vi "SMC.vi"() -> ()   [LabVIEW 2010]
doc: "This is the Superconducting Magnet Control module (SMC).\nIts job is to receive messages from the PDP, translate them into magnet commands, and send reply messages back to the PDP indicating magnet status."
uses:
  SMC Global.vi
panel:
  in  "Force Read":bool
  in  "Need to Beep":bool
  in  "Beep at Setpoint":bool=TRUE
  out "SMC Message Type":T1(ring)=enum."Ping="
  out "Magnet Entered this state at:":string
  out "Last Change":dbl format="%.2f"
  out "Update Often":bool
  out "Magnet Status":T2={"Sweep Status"=enum."To Zero", "Leads Current (A)"=0.0, "Leads Voltage (V)"=0.0, "Leads Field (T)"=0.0, "Switch Heater"=FALSE, "Setpoint (A)"=0.0, "Sweep Rate (A/min)"=0.0, "System Status"=enum."Warming Up", "Limit Status"=enum."Positive Current Limit", "Persistent Current (A)"=0.0, "Control Status"=FALSE, "Persistent Field (T)"=0.0} {"Leads Field (T)" format="%.2f"; "Persistent Field (T)" format="%.3f"; "Persistent Current (A)" format="%.3f"; "Setpoint (A)" format="%.3f"; "Leads Voltage (V)" format="%.2f"; "Sweep Rate (A/min)" format="%.2f"; "Leads Current (A)" format="%.3f"}
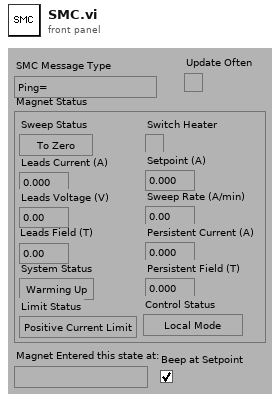
[diagram p1: front panel]
types:
  T1 = enum16{"Bad Message", "DoNothing", "Read=", "GenEvent=", "MagStatus=", "Control", "Setpoint=", "Setrate=", "Heater=", "Ping=", "Stop", "Beep"}
  T2 = cluster{"Sweep Status":enum16{"Hold", "To Setpoint", "To Zero", "Clamped"}, "Leads Current (A)":dbl, "Leads Voltage (V)":dbl, "Leads Field (T)":dbl, "Switch Heater":bool, "Setpoint (A)":dbl, "Sweep Rate (A/min)":dbl, "System Status":enum16{"Normal", "Quenched", "Over Heated", "Warming Up"}, "Limit Status":enum16{"Normal", "Positive Voltage Limit", "Negative Voltage Limit", "Negative Current Limit", "Positive Current Limit"}, "Persistent Current (A)":dbl, "Control Status":bool, "Persistent Field (T)":dbl}
  T3 = enum16{"Hold", "To Setpoint", "To Zero", "Clamped"}
  T4 = enum16{"Normal", "Quenched", "Over Heated", "Warming Up"}
  T5 = enum16{"Normal", "Positive Voltage Limit", "Negative Voltage Limit", "Negative Current Limit", "Positive Current Limit"}
  T6 = cluster{"Sweep Status":enum16{"Hold", "To Setpoint", "To Zero", "Clamped"}, "Leads Current (A)":dbl, "Leads Field (T)":dbl, "Switch Heater":bool, "Setpoint (A)":dbl, "Sweep Rate (A/min)":dbl, "System Status":enum16{"Normal", "Quenched", "Over Heated", "Warming Up"}, "Limit Status":enum16{"Normal", "Positive Voltage Limit", "Negative Voltage Limit", "Negative Current Limit", "Positive Current Limit"}, "Persistent Current (A)":dbl, "Control Status":bool, "Persistent Field (T)":dbl}
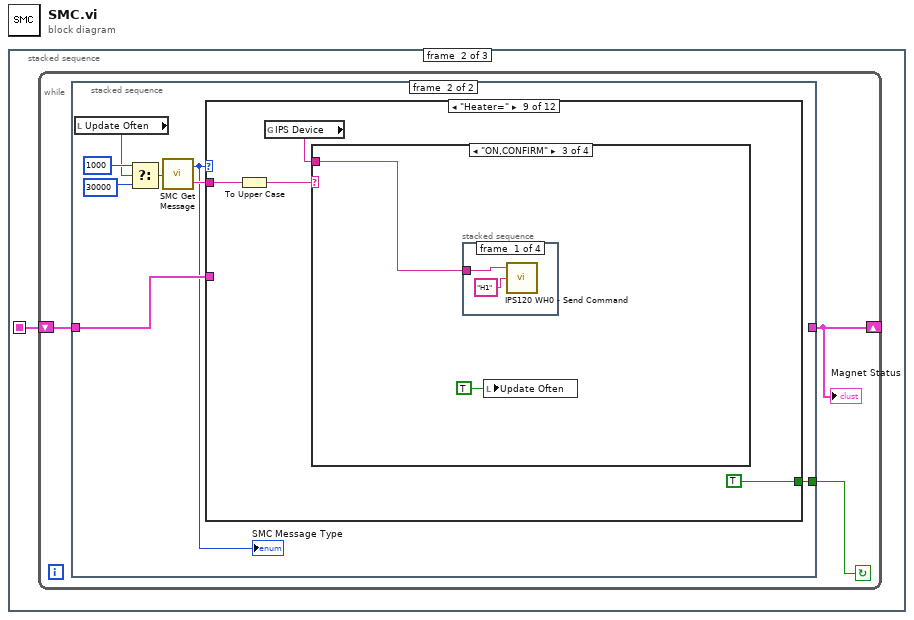
[diagram p0: block diagram]
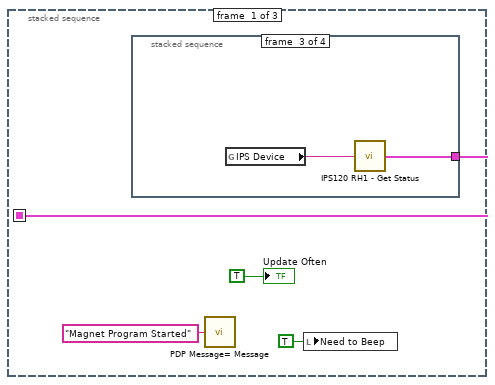
[diagram p2: hidden frame]
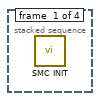
[diagram p3: hidden frame]
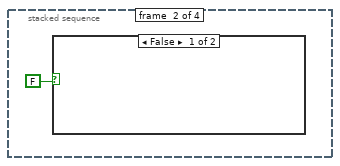
[diagram p4: hidden frame]
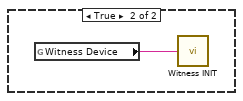
[diagram p5: hidden frame]
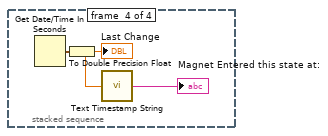
[diagram p6: hidden frame]
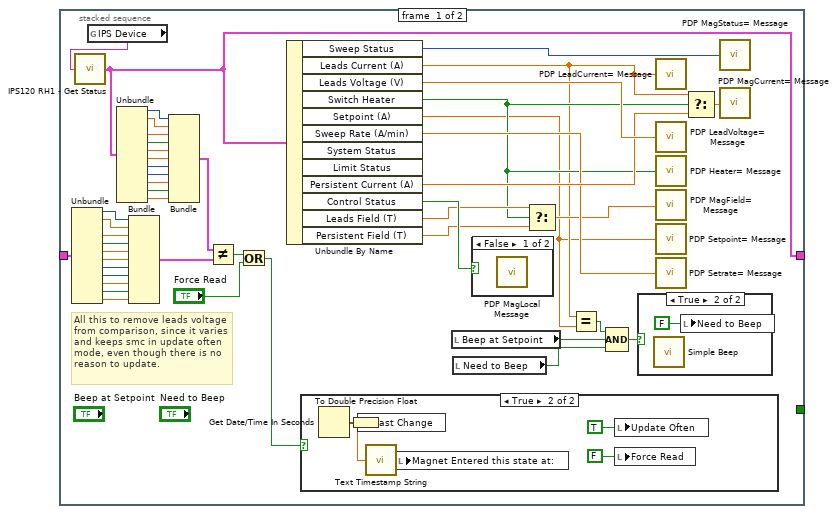
[diagram p7: hidden frame]
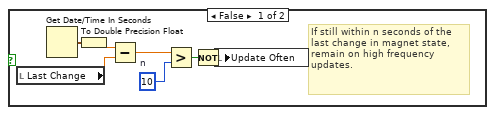
[diagram p8: hidden frame]
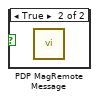
[diagram p10: hidden frame]
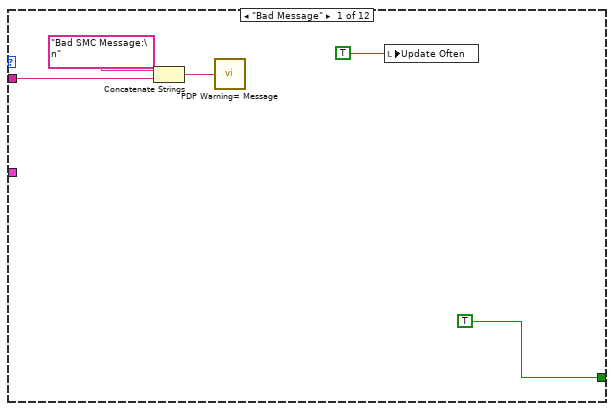
[diagram p11: hidden frame]
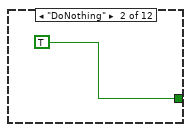
[diagram p12: hidden frame]
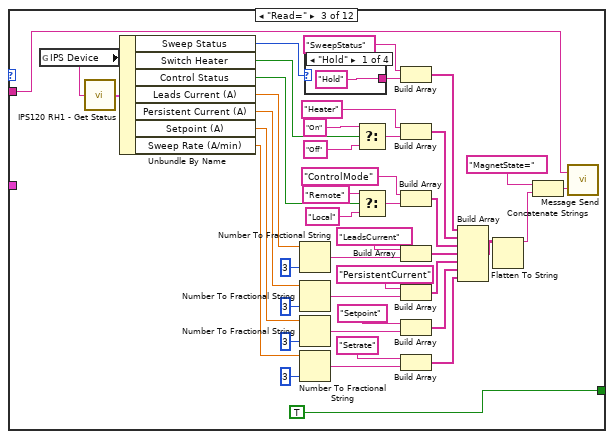
[diagram p13: hidden frame]
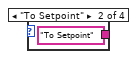
[diagram p14: hidden frame]
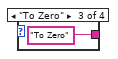
[diagram p15: hidden frame]
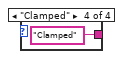
[diagram p16: hidden frame]
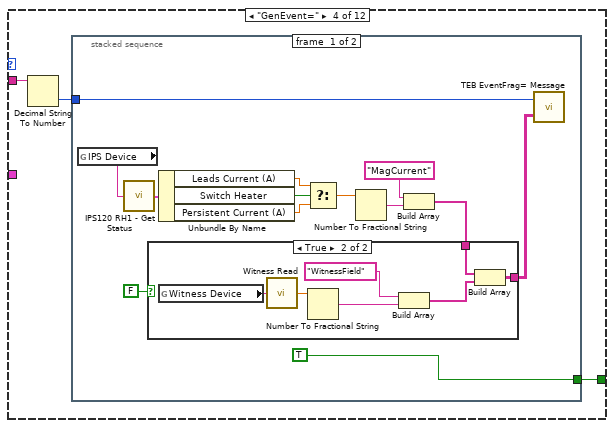
[diagram p17: hidden frame]
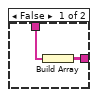
[diagram p18: hidden frame]
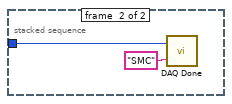
[diagram p19: hidden frame]
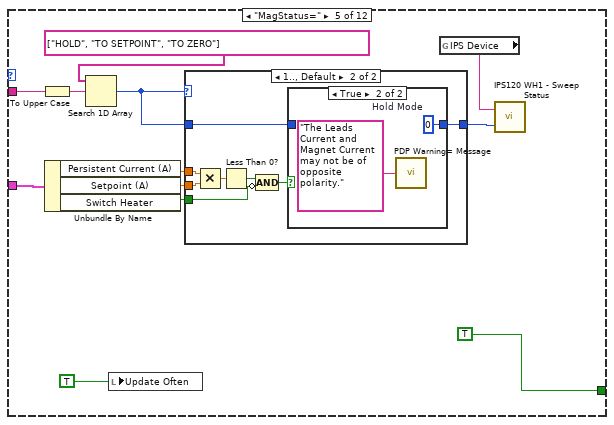
[diagram p20: hidden frame]
diagram:
  n1 = stacked-sequence {
    seq-local: [w4 _ _] -> [_ w12 _]
    frame #0 {
      n2 = stacked-sequence {
        tunnel: [_ _ w8 _] -> w4
        frame #0 {
          n3 = call "SMC INIT.vi"() -> ()  [unwired: 1 in]
        }
        frame #1 {
          n4 = case shown="False" FALSE {
            frame False {
            }
            frame True {
              n5 = global read "SMC Global.vi" "Witness Device"() -> (w6:string)
              n6 = call "Witness INIT.vi"("address string"=w6) -> ()
            }
          }
        }
        frame #2 {
          n7 = global read "SMC Global.vi" "IPS Device"() -> (w7:string)
          n8 = call "IPS120 RH1 - Get Status.vi"("GPIB Address"=w7) -> ("Magnet Status"=w8:T2)
        }
        frame #3 {
          n9 = Get Date/Time In Seconds() -> (seconds since 1Jan1904=w9:timestamp)
          n10 = To Double Precision Float(number=w9) -> (double precision float=w11:dbl)
          "Last Change" <- w11
          n11 = call "Text Timestamp String.vi"("Seconds"=w11) -> ("Timestamp String"=→"Magnet Entered this state at:":string)
        }
      }
      n12 = call "PDP Message= Message.vi"("Message"="Magnet Program Started") -> ()
      n13 = local write "Need to Beep"(TRUE ("Need to Beep")) -> ()
      "Update Often" <- TRUE ("Update Often")
    }
    frame #1 {
      n14 = while {
        shift-left: w12 -> [w14]
        shift-right: [w13] -> _
        stop <- w15 continue-if-true
        n15 = stacked-sequence {
          tunnel: [_ w81] -> w15
          tunnel: w14 -> [w60 w77]
          tunnel: [w46 _] -> w13
          frame #0 {
            # "All this to remove leads voltage from comparison, since it varies and keeps smc in update often mode, even though there is no \nreason to update."
            n16 = Unbundle(w60) -> ("Sweep Status"=w59:T3, "Leads Current (A)"=w58:dbl, "Leads Field (T)"=w57:dbl, "Switch Heater"=w56:bool, "Setpoint (A)"=w55:dbl, "Sweep Rate (A/min)"=w54:dbl, "System Status"=w53:T4, "Limit Status"=w52:T5, "Persistent Current (A)"=w43:dbl, "Control Status"=w42:bool, "Persistent Field (T)"=w41:dbl)  [unwired: 1 out]
            n17 = global read "SMC Global.vi" "IPS Device"() -> (w61:string)
            n18 = call "IPS120 RH1 - Get Status.vi"("GPIB Address"=w61) -> ("Magnet Status"=w46:T2)
            n19 = Unbundle(w46) -> ("Sweep Status"=w35:T3, "Leads Current (A)"=w36:dbl, "Leads Field (T)"=w37:dbl, "Switch Heater"=w38:bool, "Setpoint (A)"=w39:dbl, "Sweep Rate (A/min)"=w40:dbl, "System Status"=w51:T4, "Limit Status"=w50:T5, "Persistent Current (A)"=w49:dbl, "Control Status"=w48:bool, "Persistent Field (T)"=w47:dbl)  [unwired: 1 out]
            n20 = Bundle("Sweep Status"=w59, "Leads Current (A)"=w58, "Leads Field (T)"=w57, "Switch Heater"=w56, "Setpoint (A)"=w55, "Sweep Rate (A/min)"=w54, "System Status"=w53, "Limit Status"=w52, "Persistent Current (A)"=w43, "Control Status"=w42, "Persistent Field (T)"=w41) -> (w44:T6)  [unwired: 1 in]
            n21 = Bundle("Sweep Status"=w35, "Leads Current (A)"=w36, "Leads Field (T)"=w37, "Switch Heater"=w38, "Setpoint (A)"=w39, "Sweep Rate (A/min)"=w40, "System Status"=w51, "Limit Status"=w50, "Persistent Current (A)"=w49, "Control Status"=w48, "Persistent Field (T)"=w47) -> (w45:T6)  [unwired: 1 in]
            n22 = Not Equal?(x=w45, y=w44) -> (x != y?=w33:bool)
            n23 = Or(x=w33, y="Force Read") -> (x .or. y?=w16:bool)
            n24 = Unbundle By Name(w46) -> ("Sweep Status"=w32:T3, "Leads Current (A)"=w22:dbl, "Leads Voltage (V)"=w31:dbl, "Switch Heater"=w24:bool, "Setpoint (A)"=w21:dbl, "Sweep Rate (A/min)"=w28:dbl, "Persistent Current (A)"=w30:dbl, "Control Status"=w27:bool, "Leads Field (T)"=w26:dbl, "Persistent Field (T)"=w25:dbl)  [unwired: 2 out]
            n25 = case shown="True" w16 {
              frame False {
                w65 = 10  # n
                # "If still within n seconds of the last change in magnet state, remain on high frequency updates."
                n26 = local read "Last Change"() -> (w64:dbl)
                n27 = Get Date/Time In Seconds() -> (seconds since 1Jan1904=w62:timestamp)
                n28 = To Double Precision Float(number=w62) -> (double precision float=w63:dbl)
                n29 = Subtract(x=w63, y=w64) -> (x-y=w66:dbl)
                n30 = Greater?(x=w66, y=w65) -> (0:w67:bool)
                n31 = Not(x=w67) -> (.not. x?=w68:bool)
                n32 = local write "Update Often"(w68) -> ()
              }
              frame True {
                n33 = Get Date/Time In Seconds() -> (seconds since 1Jan1904=w69:timestamp)
                n34 = To Double Precision Float(number=w69) -> (double precision float=w72:dbl)
                n35 = local write "Last Change"(w72) -> ()
                n36 = call "Text Timestamp String.vi"("Seconds"=w72) -> ("Timestamp String"=w73:string)
                n37 = local write "Magnet Entered this state at:"(w73) -> ()
                n38 = local write "Update Often"(TRUE ("Update Often")) -> ()
                n39 = local write "Force Read"(FALSE ("Force Read")) -> ()
              }
            }
            n40 = local read "Beep at Setpoint"() -> (w19:bool)
            n41 = local read "Need to Beep"() -> (w18:bool)
            n42 = case shown="False" w27 {
              frame False {
                n43 = call "PDP MagLocal Message.vi"() -> ()  [unwired: 1 in]
              }
              frame True {
                n44 = call "PDP MagRemote Message.vi"() -> ()  [unwired: 1 in]
              }
            }
            n45 = Select(t=w26, s=w24, f=w25) -> (s? t:f=w23:dbl)
            n46 = Equal?(x=w22, y=w21) -> (x = y?=w20:bool)
            n47 = Compound Arithmetic op=AND(w20, w19, w18) -> (w17:bool)
            n48 = case shown="True" w17 {
              frame False {
              }
              frame True {
                n49 = call "Simple Beep.vi"() -> ()  [unwired: 1 in]
                n50 = local write "Need to Beep"(FALSE) -> ()
              }
            }
            n51 = call "PDP LeadCurrent= Message.vi"("Lead Current"=w22) -> ()
            n52 = call "PDP LeadVoltage= Message.vi"("Lead Voltage"=w31) -> ()
            n53 = call "PDP Heater= Message.vi"("Setrate"=w24) -> ()
            n54 = call "PDP MagField= Message.vi"("Mag Field"=w23) -> ()
            n55 = call "PDP Setpoint= Message.vi"("Setpoint"=w21) -> ()
            n56 = call "PDP Setrate= Message.vi"("Setrate"=w28) -> ()
            n57 = Select(t=w22, s=w24, f=w30) -> (s? t:f=w29:dbl)
            n58 = call "PDP MagStatus= Message.vi"("Mag Status"=w32) -> ()
            n59 = call "PDP MagCurrent= Message.vi"("Mag Current"=w29) -> ()
          }
          frame #1 {
            n60 = local read "Update Often"() -> (w75:bool)
            n61 = Select(t=1000, s=w75, f=30000) -> (s? t:f=w80:i32)
            n62 = call "SMC Get Message.vi"("Timeout (ms)"=w80) -> ("SMC Message Type"=w76:T1, "Text"=w82:string)
            "SMC Message Type" <- w76
            n63 = case shown="\"Heater=\"" w76 {
              tunnel: w82 -> [w87 _ w92 w138 w174 _ w196 w201 w205 w249 _ _]
              tunnel: [TRUE TRUE TRUE w139 TRUE TRUE TRUE TRUE TRUE TRUE FALSE TRUE] -> w81
              tunnel: w77 -> [_ _ _ _ w167 w191 _ _ _ _ _ _]
              frame "Bad Message" {
                n64 = Concatenate Strings("Bad SMC Message:\n", w87) -> (w85:string)
                n65 = call "PDP Warning= Message.vi"("Message"=w85) -> ()
                n66 = local write "Update Often"(TRUE) -> ()
              }
              frame "DoNothing" {
              }
              frame "Read=" {
                n67 = global read "SMC Global.vi" "IPS Device"() -> (w131:string)
                n68 = call "IPS120 RH1 - Get Status.vi"("GPIB Address"=w131) -> ("Magnet Status"=w130:T2)
                n69 = Unbundle By Name(w130) -> ("Sweep Status"=w110:T3, "Switch Heater"=w111:bool, "Control Status"=w107:bool, "Leads Current (A)"=w122:dbl, "Persistent Current (A)"=w123:dbl, "Setpoint (A)"=w124:dbl, "Sweep Rate (A/min)"=w125:dbl)
                n70 = Number To Fractional String(number=w122, precision (6)=i16 3) -> (F-format string=w121:string)  [unwired: 2 in]
                n71 = Number To Fractional String(number=w123, precision (6)=i16 3) -> (F-format string=w119:string)  [unwired: 2 in]
                n72 = Number To Fractional String(number=w124, precision (6)=i16 3) -> (F-format string=w118:string)  [unwired: 2 in]
                n73 = Number To Fractional String(number=w125, precision (6)=i16 3) -> (F-format string=w117:string)  [unwired: 2 in]
                n74 = case shown="\"Hold\"" w110 {
                  tunnel: ["Hold" "To Setpoint" "To Zero" "Clamped"] -> w102
                  frame "Hold" {
                  }
                  frame "To Setpoint" {
                  }
                  frame "To Zero" {
                  }
                  frame "Clamped" {
                  }
                }
                n75 = Select(t="On", s=w111, f="Off") -> (s? t:f=w105:string)
                n76 = Select(t="Remote", s=w107, f="Local") -> (s? t:f=w106:string)
                n77 = Build Array("SweepStatus", w102) -> (w96:string[])
                n78 = Build Array("Heater", w105) -> (w95:string[])
                n79 = Build Array("ControlMode", w106) -> (w94:string[])
                n80 = Build Array("LeadsCurrent", w121) -> (w97:string[])
                n81 = Build Array("PersistentCurrent", w119) -> (w98:string[])
                n82 = Build Array("Setpoint", w118) -> (w99:string[])
                n83 = Build Array("Setrate", w117) -> (w100:string[])
                n84 = Build Array(w96, w95, w94, w97, w98, w99, w100) -> (w93:string[][])
                n85 = Flatten To String(anything=w93) -> (data string=w90:string)  [unwired: 3 in, 2 out]
                n86 = Concatenate Strings("MagnetState=" ("Substring"), w90) -> (w91:string)
                n87 = call "Message Send.vi"("Message"=w91, "Destination"=w92) -> ()
              }
              frame "GenEvent=" {
                n88 = Decimal String To Number(string=w138) -> (number=w137:i32)  [unwired: 2 in, 1 out]
                n89 = stacked-sequence {
                  tunnel: [TRUE _] -> w139
                  tunnel: w137 -> [w151 w163]
                  frame #0 {
                    n90 = global read "SMC Global.vi" "IPS Device"() -> (w145:string)
                    n91 = call "IPS120 RH1 - Get Status.vi"("GPIB Address"=w145) -> ("Magnet Status"=w150:T2)
                    n92 = Unbundle By Name(w150) -> ("Leads Current (A)"=w143:dbl, "Switch Heater"=w144:bool, "Persistent Current (A)"=w142:dbl)
                    n93 = Select(t=w143, s=w144, f=w142) -> (s? t:f=w141:dbl)
                    n94 = Number To Fractional String(number=w141) -> (F-format string=w146:string)  [unwired: 3 in]
                    n95 = Build Array("MagCurrent", w146) -> (w148:string[])
                    n96 = case shown="True" FALSE {
                      tunnel: w148 -> [w154 w161]
                      tunnel: [w153 w160] -> w147
                      frame False {
                        n97 = Build Array(w154) -> (w153:string[][])
                      }
                      frame True {
                        n98 = global read "SMC Global.vi" "Witness Device"() -> (w155:string)
                        n99 = call "Witness Read.vi"("address string"=w155) -> ("Field"=w156:dbl)
                        n100 = Number To Fractional String(number=w156) -> (F-format string=w159:string)  [unwired: 3 in]
                        n101 = Build Array("WitnessField", w159) -> (w157:string[])
                        n102 = Build Array(w161, w157) -> (w160:string[][])
                      }
                    }
                    n103 = call "TEB EventFrag= Message.vi"("Event Fragment(s)"=w147, "Event Number"=w151) -> ()
                  }
                  frame #1 {
                    n104 = call "DAQ Done.vi"("Module Name"="SMC", "Event Number"=w163) -> ()
                  }
                }
              }
              frame "MagStatus=" {
                n105 = To Upper Case(1:w174) -> (0:w173:string)
                n106 = Unbundle By Name(w167) -> ("Persistent Current (A)"=w166:dbl, "Setpoint (A)"=w165:dbl, "Switch Heater"=w164:bool)
                n107 = Search 1D Array(1D array=string[] ["HOLD", "TO SETPOINT", "TO ZERO"], element=w173) -> (index of element=w169:i32)  [unwired: 1 in]
                n108 = local write "Update Often"(TRUE) -> ()
                n109 = case shown="1.., Default" w169 {
                  tunnel: w169 -> [w176 w181]
                  tunnel: w166 -> [_ w184]
                  tunnel: w165 -> [_ w183]
                  tunnel: [w176 w180] -> w168
                  tunnel: w164 -> [_ w178]
                  frame ..0 {
                  }
                  frame 1.., Default {
                    n110 = Multiply(x=w184, y=w183) -> (x*y=w182:dbl)
                    n111 = Less Than 0?(x=w182) -> (x < 0?=w179:bool)
                    n112 = Compound Arithmetic op=AND(w179, invert w178) -> (w177:bool)
                    n113 = case shown="True" w177 {
                      tunnel: w181 -> [w185 _]
                      tunnel: [w185 w187] -> w180
                      frame False {
                      }
                      frame True {
                        w187 = 0  # Hold Mode
                        n114 = call "PDP Warning= Message.vi"("Message"="The Leads Current and Magnet Current may not be of opposite polarity.") -> ()
                      }
                    }
                  }
                }
                n115 = global read "SMC Global.vi" "IPS Device"() -> (w172:string)
                n116 = call "IPS120 WH1 - Sweep Status.vi"("Sweep Status"=w168, "GPIB Address"=w172) -> ()
              }
              frame "Control" {
                n117 = global read "SMC Global.vi" "IPS Device"() -> (w188:string)
                n118 = Unbundle By Name(w191) -> ("Control Status"=w190:bool)
                n119 = Not(x=w190) -> (.not. x?=w189:bool)
                n120 = call "IPS120 WH4 - Remote Mode.vi"("Remote Mode"=w189, "GPIB Address"=w188) -> ()
              }
              frame "Setpoint=" {
                w193 = TRUE
                n121 = Fract/Exp String To Number(string=w196) -> (number=w195:dbl)  [unwired: 3 in, 1 out]
                n122 = global read "SMC Global.vi" "IPS Device"() -> (w194:string)
                n123 = call "IPS120 WH2 - Write Setpoint.vi"("Setpoint"=w195, "GPIB Address"=w194) -> ()
                n124 = local write "Update Often"(w193) -> ()
                n125 = local write "Need to Beep"(w193) -> ()
              }
              frame "Setrate=" {
                n126 = Fract/Exp String To Number(string=w201) -> (number=w200:dbl)  [unwired: 3 in, 1 out]
                n127 = global read "SMC Global.vi" "IPS Device"() -> (w199:string)
                n128 = call "IPS120 WH3 - Write Setrate.vi"("Setrate"=w200, "GPIB Address"=w199) -> ()
                n129 = local write "Update Often"(TRUE) -> ()
              }
              frame "Heater=" {
                n130 = To Upper Case(1:w205) -> (0:w203:string)
                n131 = global read "SMC Global.vi" "IPS Device"() -> (w204:string)
                n132 = case shown="\"ON,CONFIRM\"" w203 {
                  tunnel: w204 -> [w208 w218 w233 w240]
                  frame "OFF", Default {
                    n133 = call "IPS120 RH1 - Get Status.vi"("GPIB Address"=w208) -> ("Magnet Status"=w207:T2)
                    n134 = stacked-sequence {
                      tunnel: w208 -> [w211 _ _]
                      tunnel: w207 -> [_ w213 _]
                      frame #0 {
                        n135 = call "IPS120 WH0 - Send Command.vi"("Command String"="H0", "VISA Address"=w211) -> ()  [unwired: 1 in, 3 out]
                      }
                      frame #1 {
                        # "If heater was on, wait 30 sec for it to go off."
                        n136 = Unbundle By Name(w213) -> ("Switch Heater"=w212:bool)
                        n137 = case shown="True" w212 {
                          frame False {
                          }
                          frame True {
                            n138 = stacked-sequence {
                              frame #0 {
                                n139 = call "PDP HeaterDelay= Message.vi"("Setrate"=i8 30 ("Heater Delay (sec)")) -> ()
                              }
                              frame #1 {
                                n140 = Wait (ms)(milliseconds to wait=u32 30000) -> ()  [unwired: 1 out]
                              }
                            }
                          }
                        }
                      }
                      frame #2 {
                        n141 = call "PDP Heater= Message.vi"("Setrate"=FALSE ("Switch Heater")) -> ()
                      }
                    }
                    n142 = local write "Update Often"(TRUE) -> ()
                  }
                  frame "ON" {
                    n143 = call "IPS120 RH1 - Get Status.vi"("GPIB Address"=w218) -> ("Magnet Status"=w225:T2)
                    n144 = Unbundle By Name(w225) -> ("Sweep Status"=w223:T3, "Leads Current (A)"=w222:dbl, "Persistent Current (A)"=w221:dbl)
                    n145 = Equal?(x=T3."Hold" ("Sweep Status"), y=w223) -> (x = y?=w217:bool)
                    n146 = Equal?(x=w222, y=w221) -> (x = y?=w219:bool)
                    n147 = Compound Arithmetic op=AND(w217, w219) -> (w220:bool)
                    n148 = case shown="True" w220 {
                      tunnel: w219 -> [w229 _]
                      tunnel: w218 -> [_ _]
                      frame False {
                        n149 = Select(t="The Magnet Power Supply needs to be in Hold Mode.", s=w229, f="The Magnet Leads do not match the current in the magnet.") -> (s? t:f=w226:string)
                        n150 = call "PDP Warning= Message.vi"("Message"=w226) -> ()
                      }
                      frame True {
                        n151 = call "Message Send.vi"("Message"="HeaterDialog", "Destination"="PDP") -> ()
                      }
                    }
                  }
                  frame "ON,CONFIRM" {
                    n152 = stacked-sequence {
                      tunnel: w233 -> [w235 _ _ _]
                      frame #0 {
                        n153 = call "IPS120 WH0 - Send Command.vi"("Command String"="H1", "VISA Address"=w235) -> ()  [unwired: 1 in, 3 out]
                      }
                      frame #1 {
                        n154 = call "PDP HeaterDelay= Message.vi"("Setrate"=i8 30 ("Heater Delay (sec)")) -> ()
                      }
                      frame #2 {
                        n155 = Wait (ms)(milliseconds to wait=u32 30000) -> ()  [unwired: 1 out]
                      }
                      frame #3 {
                        n156 = call "PDP Heater= Message.vi"("Setrate"=TRUE ("Switch Heater")) -> ()
                      }
                    }
                    n157 = local write "Update Often"(TRUE) -> ()
                  }
                  frame "ON,FORCE" {
                    n158 = stacked-sequence {
                      tunnel: w240 -> [w242 _ _ _]
                      frame #0 {
                        n159 = call "IPS120 WH0 - Send Command.vi"("Command String"="H1", "VISA Address"=w242) -> ()  [unwired: 1 in, 3 out]
                      }
                      frame #1 {
                        n160 = call "PDP HeaterDelay= Message.vi"("Setrate"=i8 30 ("Heater Delay (sec)")) -> ()
                      }
                      frame #2 {
                        n161 = Wait (ms)(milliseconds to wait=u32 30000) -> ()  [unwired: 1 out]
                      }
                      frame #3 {
                        n162 = call "PDP Heater= Message.vi"("Setrate"=TRUE ("Switch Heater")) -> ()
                      }
                    }
                    n163 = local write "Update Often"(TRUE) -> ()
                  }
                }
              }
              frame "Ping=" {
                n164 = Get Date/Time In Seconds() -> (seconds since 1Jan1904=w246:timestamp)
                n165 = To Double Precision Float(number=w246) -> (double precision float=w251:dbl)
                n166 = Format Into String(format string="PingResponse=SMC,%.0f", w251) -> (resulting string=w252:string)  [unwired: 2 in, 1 out]
                n167 = call "Message Send.vi"("Message"=w252, "Destination"=w249) -> ()
                n168 = local write "Update Often"(TRUE ("Update Often")) -> ()
              }
              frame "Stop" {
              }
              frame "Beep" {
                n169 = call <vilib>:"Beep.vi"() -> ()  [unwired: 12 in]
              }
            }
          }
        }
        "Magnet Status" <- w13
      }
    }
    frame #2 {
    }
  }
